vi "setAngle.vi"(6 "Channel":i32, 8 "error in (no error)":errorcluster, 9 "Rate (°/min)":dbl, 10 "Angle (°)":dbl, 11 "Instrument.Cryostat in":refnum<class "Instrument.Cryostat.lvclass">) -> (0 "error out":errorcluster, 3 "Instrument.Cryostat out":refnum<class "Instrument.Cryostat.lvclass">)   [LabVIEW 2019, in "Instrument.Cryostat.lvclass"]
uses:
  Instrument.Cryostat.lvclass
  Typedefs/setAngle--cluster.ctl
  769e9fe3-7829-4201-aff9-72d4f9064154.vi
  Typedefs/Cryostat.commands--enum.ctl
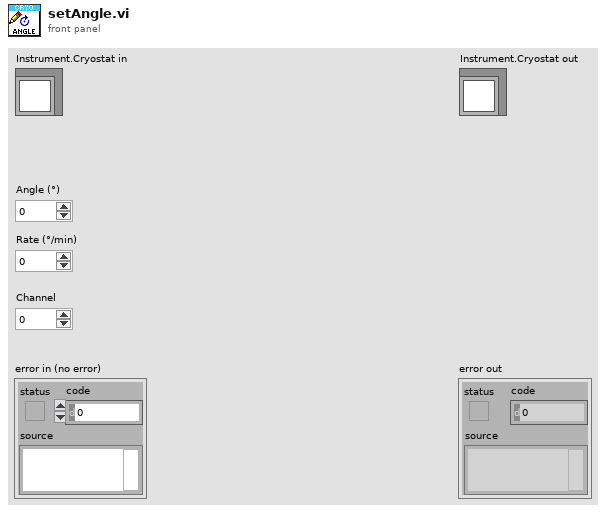
[diagram p1: front panel]
types:
  T1 = typedef "Instrument.Cryostat.lvclass/Cryostat.commands--enum.ctl" = enum16{"getLN2Level", "getLHeLevel", "getMagnet", "getMagnetVector", "setMagnet", "setMagnetVector", "getAngle", "setAngle", "getTemperature", "setTemperature", "getHeater", "setHeater", "getChamber", "setChamber", ""}
  T2 = typedef "Instrument.Cryostat.lvclass/setAngle--cluster.ctl" = cluster{"angle":dbl, "rate":dbl, "channel":i32}
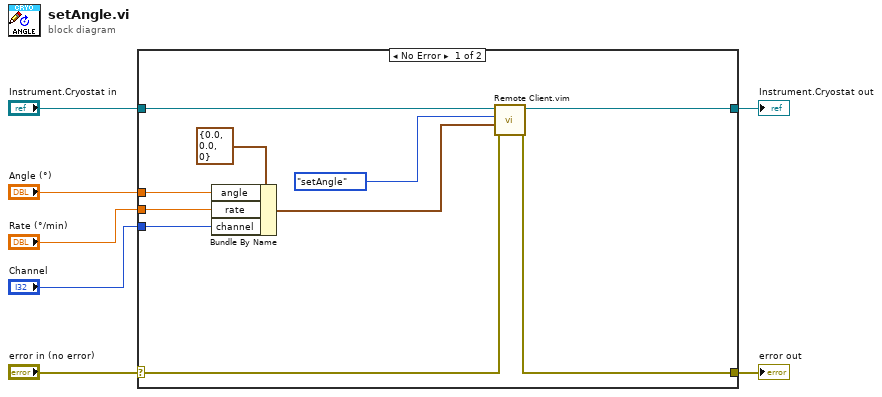
[diagram p0: block diagram]
diagram:
  n1 = case shown="No Error" "error in (no error)" {
    selector: "error in (no error)" -> [w8 w19]
    tunnel: [w12 w19] -> w6
    tunnel: [w13 w18] -> w4
    tunnel: "Instrument.Cryostat in" -> [w9 w18]
    tunnel: "Angle (°)" -> [w16 _]
    tunnel: "Rate (°/min)" -> [w15 _]
    tunnel: "Channel" -> [w14 _]
    frame No Error {
      n2 = Bundle By Name(cluster=T2 {"angle"=0.0, "rate"=0.0, "channel"=0} ("Set Angle"), "angle"=w16, "rate"=w15, "channel"=w14) -> (w11:T2)
      n3 = call "Remote Client.vim"("error in (no error)"=w8, "Data in"=w11, "Command in"=Cryostat.commands--enum."setAngle" ("commands"), "Instrument in"=w9) -> ("error out"=w12:errorcluster, "Instrument out"=w13:refnum<class "Instrument.Cryostat.lvclass">)  [unwired: 4 in, 2 out]
    }
    frame Error {
    }
  }
  "error out" <- w6
  "Instrument.Cryostat out" <- w4
